vi "Drive Global.vi"() -> ()   [LabVIEW 2013]
panel:
  in  "Slow to":dbl
  in  "Dead Band Value":dbl
  in  "Drive Info":T1
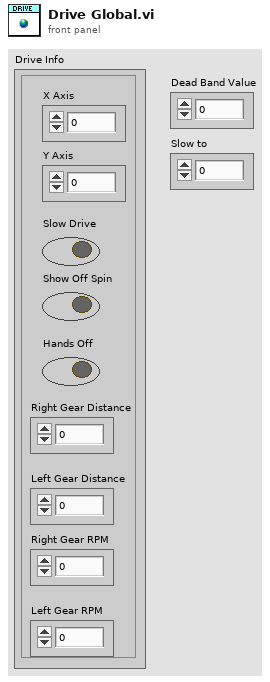
[diagram p1: front panel]
types:
  T1 = cluster{"X Axis":dbl, "Y Axis":dbl, "Slow Drive":bool, "Show Off Spin":bool, "Hands Off":bool, "Right Gear Distance":dbl, "Left Gear Distance ":dbl, "Right Gear RPM":dbl, "Left Gear RPM":dbl}
diagram:
